vi "Is_TestDataInSpec-1组数据不同规格 -角度判断共用规格.vi"(0 "相机量测结果":dbl[](array[numeric]), 1 "量测规格数组 in":T1[](array[typedef]) {"上限" format="%#.4g"; "下限" format="%#.4g"}) -> (3 "在规格内":bool, 4 "相机量测结果 out":dbl[](array[numeric]), 5 "数组":bool[](array[boolean]))   [LabVIEW 2014]
uses:
  Controls/TestThreshold.ctl
panel:
  # "~"
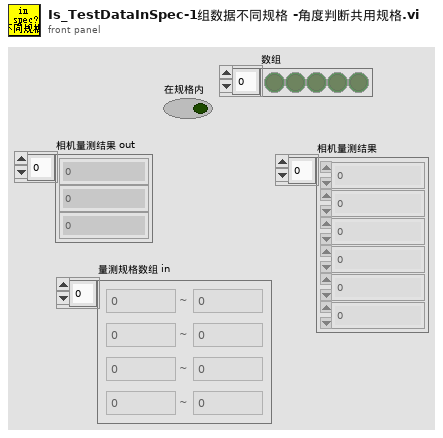
[diagram p1: front panel]
types:
  T1 = typedef "TestThreshold.ctl" = cluster{"下限":dbl, "上限":dbl}
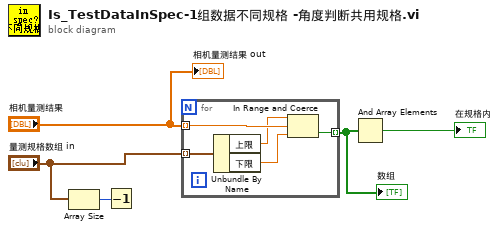
[diagram p0: block diagram]
diagram:
  n1 = Array Size(array="量测规格数组 in") -> (size(s)=w1:i32)
  n2 = Decrement(x=w1) -> ()  [unwired: 1 out]
  n3 = for {
    tunnel: "相机量测结果" -> [w10] mode=indexing
    tunnel: [w7] -> w4 mode=indexing
    tunnel: "量测规格数组 in" -> [w6] mode=indexing
    n4 = Unbundle By Name(w6) -> ("上限"=w8:dbl, "下限"=w9:dbl)
    n5 = In Range and Coerce(upper limit=w8, x=w10, lower limit=w9) -> (In Range?=w7:bool)  [unwired: 1 out]
  }
  "数组" <- w4
  n6 = And Array Elements(Boolean array=w4) -> (logical AND=→"在规格内":bool)
  "相机量测结果 out" <- "相机量测结果"
